vi "Correct Temperature.vi"(7 "Cal LUT":dbl[][][](array[numeric]), 8 "Divider Ratio":dbl, 9 "TC Channel Config":T1 {"Temperature Units" items=["Celcius", "Fahrenheit", "Kelvin", "Rankine", "Volts"]; "Thermocouple Type" items=["J", "K", "T", "E", "N", "B", "R", "S", "Raw Voltage"]}, 10 "CJC":dbl, 11 "Rquested Output Temp":dbl) -> (2 "Corrected Output Temp":dbl, 3 "Voltage Out":dbl)   [LabVIEW 2011, in "Simulated Thermocouple Custom Device.lvlib"]
uses:
  Simulated Thermocouple Custom Device.lvlib
  TC Channel Config Data.ctl
  TC Selector.ctl
  TC Unit Selector.ctl
  <vilib>/gmath/NI_Gmath.lvlib
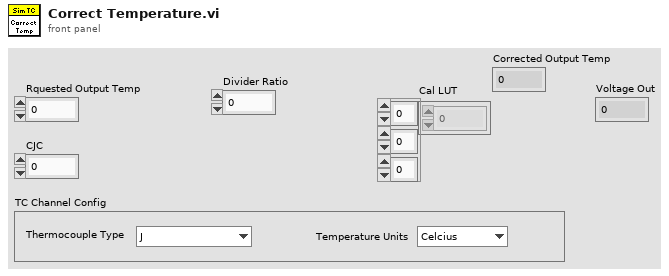
[diagram p1: front panel]
types:
  T1 = typedef "Simulated Thermocouple Custom Device.lvlib/TC Channel Config Data.ctl" = cluster{"Thermocouple Type":T2, "Temperature Units":T3}
  T2 = typedef "Simulated Thermocouple Custom Device.lvlib/TC Selector.ctl" = u16
  T3 = typedef "Simulated Thermocouple Custom Device.lvlib/TC Unit Selector.ctl" = u16
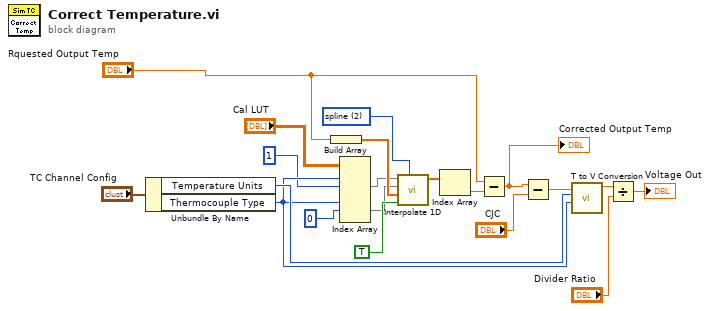
[diagram p0: block diagram]
diagram:
  w13 = 2 items=["nearest", "linear", "spline", "cubic Hermite", "Lagrange"] ("method")
  n1 = Unbundle By Name("TC Channel Config") -> ("Temperature Units"=w20:T3, "Thermocouple Type"=w14:T2)
  n2 = Build Array("Rquested Output Temp") -> (w11:dbl[])
  n3 = Index Array(array="Cal LUT", index (dim 0) #1=w14, index (dim 1) #1=1 ("disabled index (col)"), index (dim 0) #2=w14, index (dim 1) #2=0 ("index (col)")) -> (element #1=w6:dbl[], element #2=w5:dbl[])  [unwired: 2 in]
  n4 = call <vilib>:"Interpolate 1D.vi"("method"=w13, "X is monotonic"=TRUE, "xi"=w11, "X"=w5, "Y"=w6) -> ("yi"=w10:dbl[])  [unwired: 4 in, 2 out]
  n5 = Index Array(array=w10) -> (element=w9:dbl)  [unwired: 1 in]
  n6 = Subtract(x="Rquested Output Temp", y=w9) -> (x-y=w4:dbl)
  "Corrected Output Temp" <- w4
  n7 = Subtract(x=w4, y="CJC") -> (x-y=w1:dbl)
  n8 = call "T to V Conversion.vi"("Thermocouple Type"=w14, "Temperature Units"=w20, "Temperature"=w1) -> ("Voltage Out"=w18:dbl)  [unwired: 8 in]
  n9 = Divide(x=w18, y="Divider Ratio") -> (x/y=→"Voltage Out":dbl)
